vi "MGCC_FntStaMach_Visitualization_OpalRT_demo.vi"() -> ()   [LabVIEW 2016]
panel:
  out "3":cluster{dbl[], dbl[]}(graph)
  in  "S1011-STATUS-CTRL":dbl
  in  "S0910-STATUS-CTRL":dbl
  in  "S0709-STATUS-CTRL":dbl
  in  "S0708-STATUS-CTRL":dbl
  in  "S0405-STATUS-CTRL":dbl
  in  "S0307-STATUS-CTRL":dbl
  in  "S0304-STATUS-CTRL":dbl
  in  "S0203-STATUS-CTRL":dbl
  out "7":cluster{dbl[], dbl[]}(graph)
  out "10":cluster{dbl[], dbl[]}(graph)
  out "13":cluster{dbl[], dbl[]}(graph)
  out "14":cluster{dbl[], dbl[]}(graph)
  out "6":cluster{dbl[], dbl[]}(graph)
  out "1":cluster{dbl[], dbl[]}(graph)
  in  "Tab Control 2":T1(tab)
  out "Loads Power":dbl(graph)
  out "Loads Power":dbl(graph)
  out "Loads Power":dbl(graph)
  out "Loads Power":dbl(graph)
  out "Loads Power":dbl(graph)
  out "Loads Power":dbl(graph)
  out "Loads Power":dbl(graph)
  out "Loads Power":dbl(graph)
  out "Loads Power":dbl(graph)
  in  "Tab Control":T1(tab)
  out "Voltage":dbl(graph)
  out "Voltage":dbl(graph)
  out "Voltage":dbl(graph)
  out "Voltage":dbl(graph)
  out "Voltage":dbl(graph)
  out "Voltage":dbl(graph)
  out "Voltage":dbl(graph)
  out "Voltage":dbl(graph)
  out "Voltage":dbl(graph)
  out "Data Acquisition":bool
  out "Reactive power control":bool
  out "Active power control":bool
  out "Resynchronization":bool
  out "Communication":bool
  out "Data Acquisition":bool
  out "Reactive power control":bool
  out "Active power control":bool
  out "Resynchronization":bool
  out "Communication":bool
  in  "Island 3":bool
  in  "Island 2":bool
  in  "Island":bool
  in  "Ready for STD":bool
  in  "Recon cmd":bool
  in  "BKS cmd":bool
  in  "island cmd":bool
  out "Angle Difference 4":dbl
  out "Angle Difference 3":dbl
  out "Angle Difference 2":dbl
  out "Angle Difference 1":dbl
  out "BESS LC":bool
  out "PV LC":bool
  out "Model Mgmt.":bool
  out "PV Forecasting":bool
  out "Load Forecasting":bool
  out "PQ Balance":bool
  out "Black Start":bool
  out "Data Logging":bool
  out "Communication":bool
  out "State Estimation":bool
  out "Energy Mgmt.":bool
  out "SOC Tank":dbl(slide) scale=0.0..1.0
  out "S1114":bool
  out "S1011":bool
  out "S1012":bool
  out "S1013":bool
  out "S0910":bool
  out "S0708":bool
  out "S0709":bool
  out "S0307":bool
  out "S0304":bool
  out "S0406":bool
  out "S0405":bool
  out "S0203":bool
  out "S0102":bool
  out "W11":bool
  out "W13":bool
  out "W5":bool
  out "W8":bool
  out "L11":bool
  out "W12":bool
  out "L10":bool
  out "L7":bool
  out "L9":bool
  out "W7":bool
  out "W14":bool
  out "L8":bool
  out "L4":bool
  out "L5":bool
  out "W6":bool
  out "W3":bool
  out "L3":bool
  out "W2":bool
  out "L2":bool
  out "W1":bool
  out "Battery Output":dbl format="%#_6f"
  out "Battery SOC":dbl format="%#_6f"
  in  "PV-12":dbl(slide) scale=0.0..2.0
  out "PV Power Output":dbl format="%#_6f"
  out "PV Forecast":dbl[](graph)
  out "W4":bool
  out "Current State":string
  out "Sources Power":T2(graph)
  out "Frequency":T3(graph)
  out "W9":bool
  # "Title"
  # "G-6"
  # "Microgrid Local\nController 1"
  # "G-14"
  # "Microgrid Local\nController 2"
  # "Microgrid Central\nController"
  # "G-1"
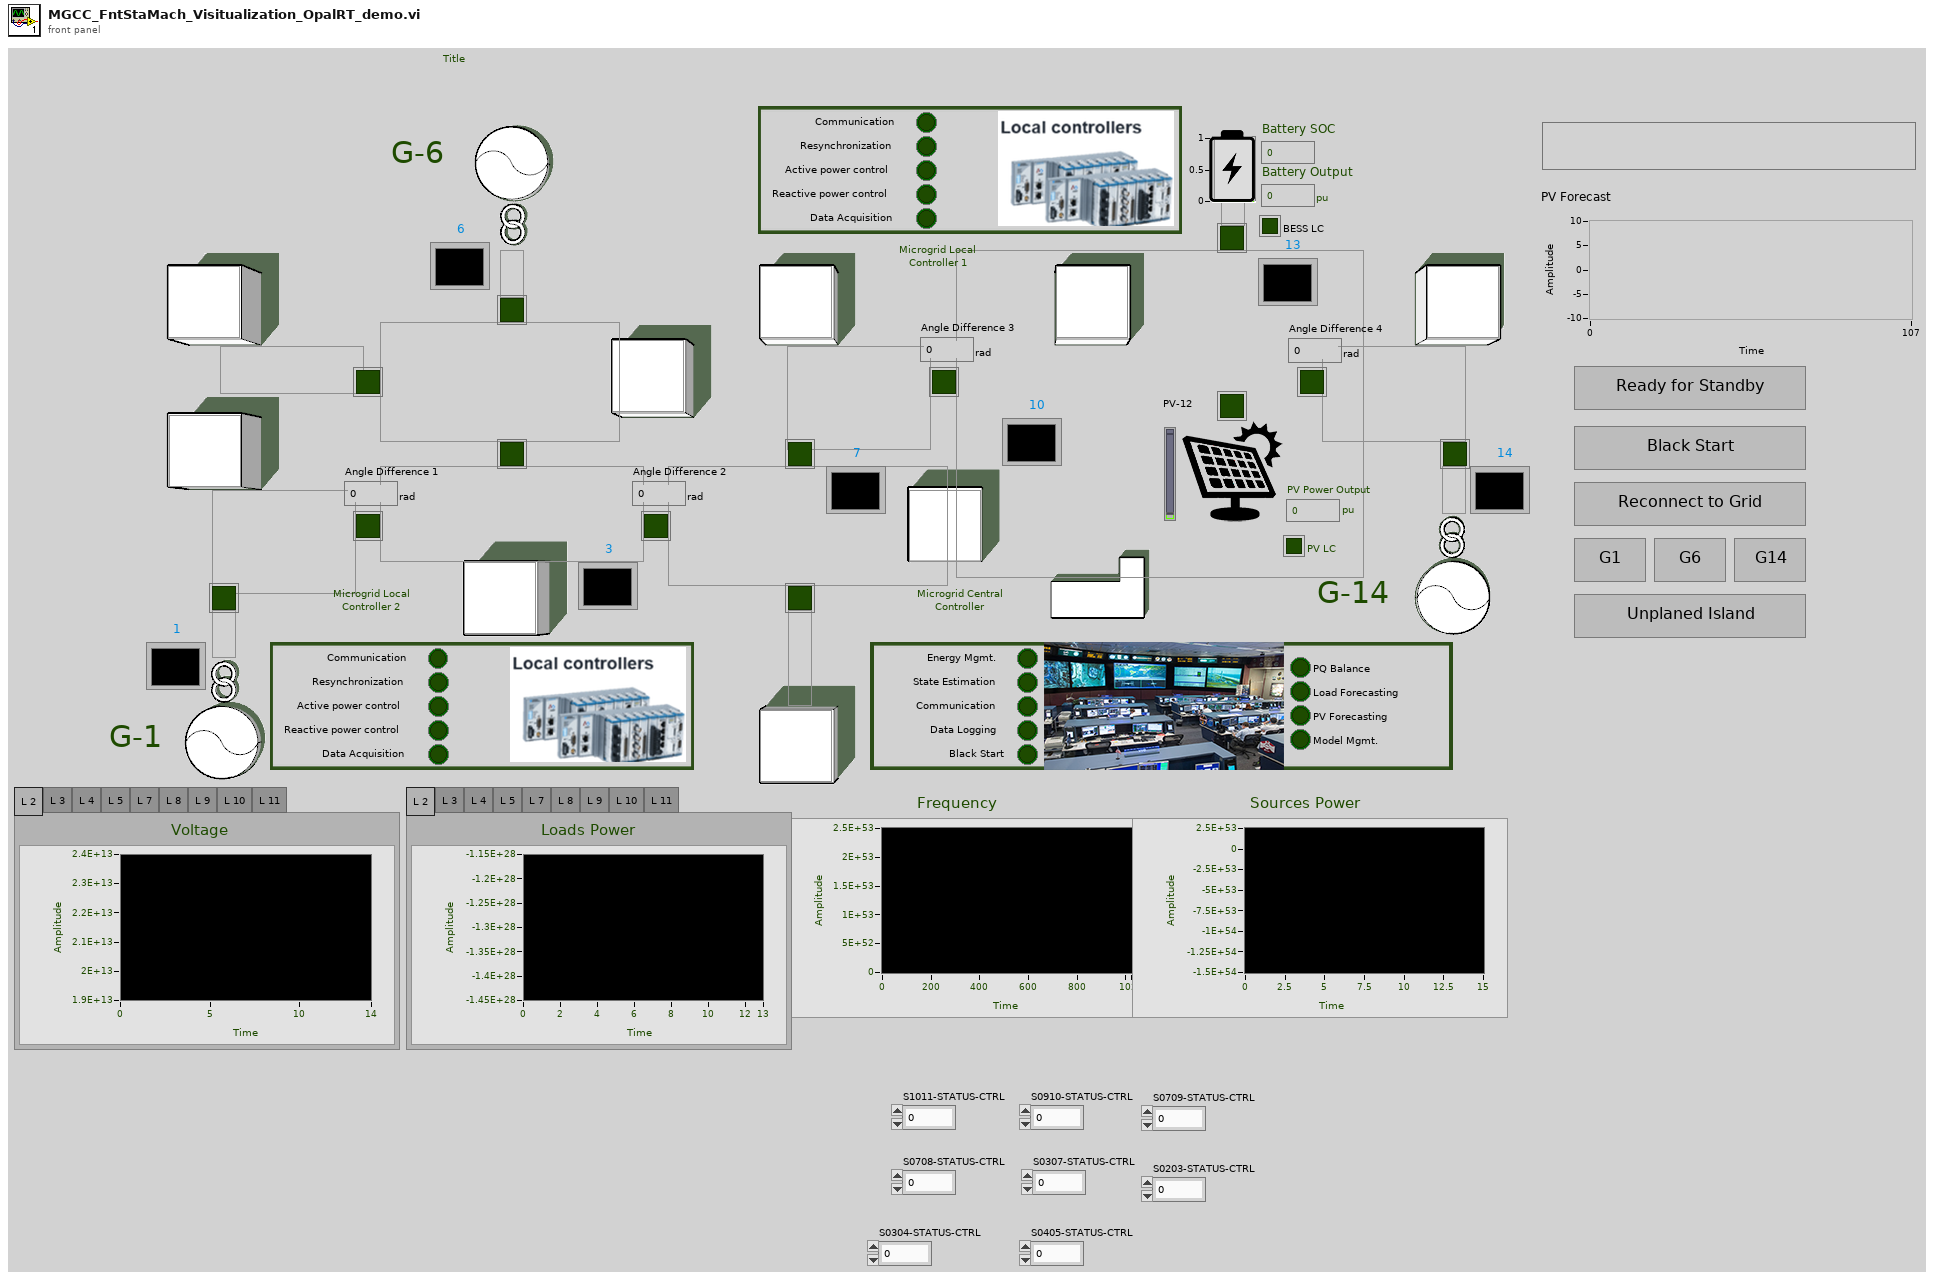
[diagram p1: front panel]
types:
  T1 = enum32{"L 2", "L 3", "L 4", "L 5", "L 7", "L 8", "L 9", "L 10", "L 11"}
  T2 = cluster{"Double":dbl, "Double":dbl, "Double":dbl, "Double":dbl, "Double":dbl}
  T3 = cluster{"Double":dbl, "Double":dbl, "Double":dbl, "Double":dbl}
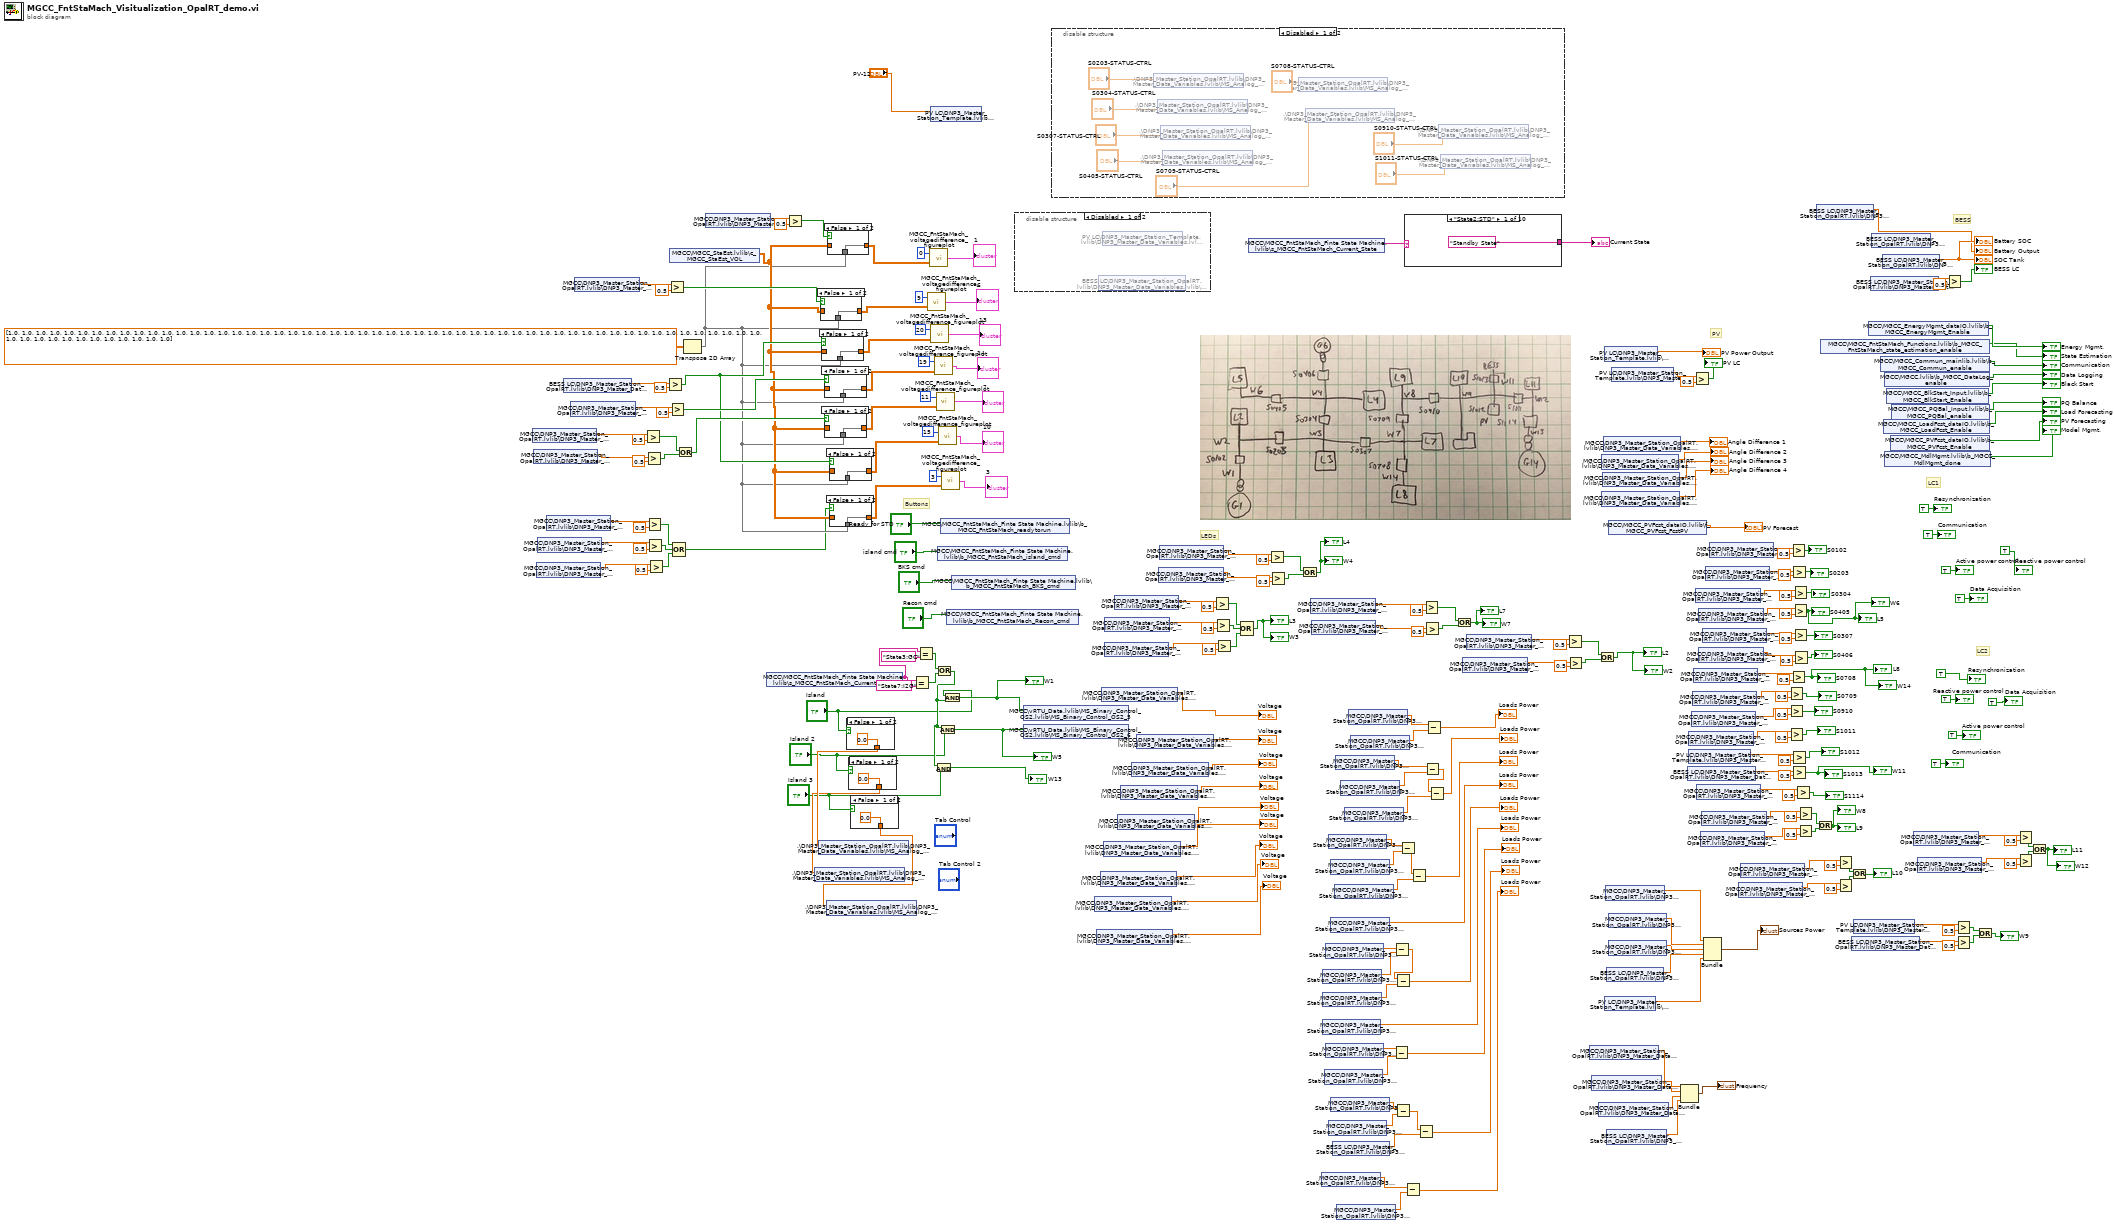
[diagram p0: block diagram]
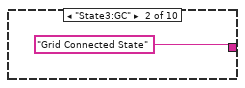
[diagram p2: hidden frame]
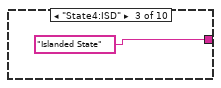
[diagram p3: hidden frame]
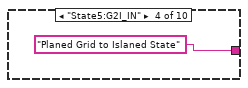
[diagram p4: hidden frame]
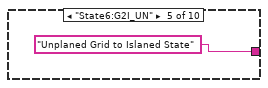
[diagram p5: hidden frame]
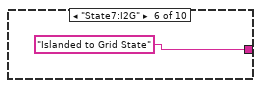
[diagram p6: hidden frame]
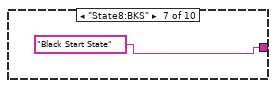
[diagram p7: hidden frame]
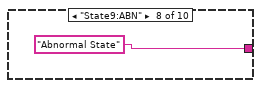
[diagram p8: hidden frame]
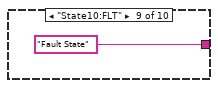
[diagram p9: hidden frame]
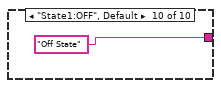
[diagram p10: hidden frame]
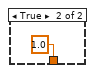
[diagram p12: hidden frame]
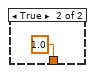
[diagram p13: hidden frame]
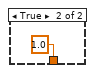
[diagram p14: hidden frame]
diagram:
  # "LC1"
  # "LC2"
  # "PV"
  # "BESS"
  # "Buttons"
  # "LEDs"
  n1 = shared-variable "MGCC\\DNP3_Master_Station_OpalRT.lvlib\\DNP3_Master_Data_Variables.lvlib\\MS_Analog_Status.lvlib\\S0307-status"() -> (w29:dbl)  [unwired: 1 in, 1 out]
  n2 = shared-variable "MGCC\\DNP3_Master_Station_OpalRT.lvlib\\DNP3_Master_Data_Variables.lvlib\\MS_Analog_Status.lvlib\\S0709-status"() -> (w28:dbl)  [unwired: 1 in, 1 out]
  n3 = shared-variable "MGCC\\DNP3_Master_Station_OpalRT.lvlib\\DNP3_Master_Data_Variables.lvlib\\MS_Analog_Status.lvlib\\S0307-status"() -> (w15:dbl)  [unwired: 1 in, 1 out]
  n4 = shared-variable "MGCC\\DNP3_Master_Station_OpalRT.lvlib\\DNP3_Master_Data_Variables.lvlib\\MS_Analog_Status.lvlib\\S0304-status"() -> (w16:dbl)  [unwired: 1 in, 1 out]
  n5 = shared-variable "MGCC\\DNP3_Master_Station_OpalRT.lvlib\\DNP3_Master_Data_Variables.lvlib\\MS_Analog_Status.lvlib\\S0203-status"() -> (w17:dbl)  [unwired: 1 in, 1 out]
  n6 = shared-variable "BESS LC\\DNP3_Master_Station_OpalRT.lvlib\\DNP3_Master_Data_Variables.lvlib\\MS_Analog_Status.lvlib\\BESS-STATUS"() -> (w41:dbl)  [unwired: 1 in, 1 out]
  n7 = shared-variable "MGCC\\DNP3_Master_Station_OpalRT.lvlib\\DNP3_Master_Data_Variables.lvlib\\MS_Analog_Status.lvlib\\S1114-status"() -> (w35:dbl)  [unwired: 1 in, 1 out]
  n8 = shared-variable "MGCC\\DNP3_Master_Station_OpalRT.lvlib\\DNP3_Master_Data_Variables.lvlib\\MS_Analog_Status.lvlib\\S0406-status"() -> (w44:dbl)  [unwired: 1 in, 1 out]
  n9 = Greater?(x=w29, y=0.5) -> (0:w31:bool)
  n10 = Greater?(x=w28, y=0.5) -> (0:w30:bool)
  n11 = Greater?(x=w17, y=0.5) -> (0:w14:bool)
  n12 = Greater?(x=w16, y=0.5) -> (0:w13:bool)
  n13 = Greater?(x=w15, y=0.5) -> (0:w12:bool)
  n14 = Greater?(x=w41, y=0.5) -> (0:w26:bool)
  n15 = Greater?(x=w44, y=0.5) -> (0:w43:bool)
  n16 = Greater?(x=w35, y=0.5) -> (0:w34:bool)
  n17 = shared-variable "MGCC\\MGCC_StaEst.lvlib\\c_MGCC_StaEst_VOL"() -> (w22:cdb[][])  [unwired: 1 in, 1 out]
  n18 = Compound Arithmetic op=OR(w14, w13, w12) -> (w11:bool)
  n19 = Or(x=w31, y=w30) -> (x .or. y?=w27:bool)
  n20 = Transpose 2D Array(2D array=dbl[][] [[1.0, 1.0, 1.0, 1.0, 1.0, 1.0, 1.0, 1.0, 1.0, 1.0, 1.0, 1.0, 1.0, 1.0, 1.0, 1.0, 1.0, 1.0, 1.0, 1.0, 1.0, 1.0], [1.0, 1.0, 1.0, 1.0, 1.0, 1.0, 1.0, 1.0, 1.0, 1.0, 1.0, 1.0, 1.0, 1.0, 1.0, 1.0, 1.0, 1.0, 1.0, 1.0, 1.0, 1.0], [1.0, 1.0, 1.0, 1.0, 1.0, 1.0, 1.0, 1.0, 1.0, 1.0, 1.0, 1.0, 1.0, 1.0, 1.0, 1.0, 1.0, 1.0, 1.0, 1.0, 1.0, 1.0]] ("lower limit")) -> (transposed array=w21:dbl[][])
  n21 = shared-variable "MGCC\\DNP3_Master_Station_OpalRT.lvlib\\DNP3_Master_Data_Variables.lvlib\\MS_Analog_Status.lvlib\\S0102-status"() -> (w48:dbl)  [unwired: 1 in, 1 out]
  n22 = shared-variable "MGCC\\MGCC_FntStaMach_Finte State Machine.lvlib\\s_MGCC_FntStaMach_Current_State"() -> (w64:string)  [unwired: 1 in, 1 out]
  n23 = Greater?(x=w48, y=0.5) -> (0:w47:bool)
  n24 = case shown="False" w43 {
    tunnel: w22 -> [_ w259]
    tunnel: [w258 w259] -> w46
    tunnel: w21 -> [w258 _]
    frame False {
    }
    frame True {
    }
  }
  n25 = case shown="False" w26 {
    tunnel: w22 -> [_ w261]
    tunnel: [w260 w261] -> w40
    tunnel: w21 -> [w260 _]
    frame False {
    }
    frame True {
    }
  }
  n26 = case shown="False" w34 {
    tunnel: w22 -> [_ w263]
    tunnel: [w262 w263] -> w39
    tunnel: w21 -> [w262 _]
    frame False {
    }
    frame True {
    }
  }
  n27 = case shown="False" w27 {
    tunnel: w22 -> [_ w265]
    tunnel: [w264 w265] -> w38
    tunnel: w21 -> [w264 _]
    frame False {
    }
    frame True {
    }
  }
  n28 = case shown="False" w47 {
    tunnel: w22 -> [_ w267]
    tunnel: [w266 w267] -> w50
    tunnel: w21 -> [w266 _]
    frame False {
    }
    frame True {
    }
  }
  n29 = case shown="False" w26 {
    tunnel: w22 -> [_ w269]
    tunnel: [w268 w269] -> w37
    tunnel: w21 -> [w268 _]
    frame False {
    }
    frame True {
    }
  }
  n30 = case shown="False" w11 {
    tunnel: w22 -> [_ w271]
    tunnel: [w270 w271] -> w23
    tunnel: w21 -> [w270 _]
    frame False {
    }
    frame True {
    }
  }
  n31 = case shown="False" "Island" {
    tunnel: [0.0 1.0] -> w8
    frame False {
    }
    frame True {
    }
  }
  n32 = shared-variable ".\\DNP3_Master_Station_OpalRT.lvlib\\DNP3_Master_Data_Variables.lvlib\\MS_Analog_Control.lvlib\\S0102-STATUS-CTRL"(w8) -> ()  [unwired: 1 in, 1 out]
  n33 = case shown="False" "Island 2" {
    tunnel: [0.0 1.0] -> w6
    frame False {
    }
    frame True {
    }
  }
  n34 = shared-variable ".\\DNP3_Master_Station_OpalRT.lvlib\\DNP3_Master_Data_Variables.lvlib\\MS_Analog_Control.lvlib\\S0406-STATUS-CTRL"(w6) -> ()  [unwired: 1 in, 1 out]
  n35 = case shown="False" "Island 3" {
    tunnel: [0.0 1.0] -> w4
    frame False {
    }
    frame True {
    }
  }
  n36 = shared-variable ".\\DNP3_Master_Station_OpalRT.lvlib\\DNP3_Master_Data_Variables.lvlib\\MS_Analog_Control.lvlib\\S1114-STATUS-CTRL"(w4) -> ()  [unwired: 1 in, 1 out]
  n37 = Equal?(x=w64, y="State7:I2G") -> (x = y?=w229:bool)
  n38 = Equal?(x=w64, y="State3:GC") -> (x = y?=w228:bool)
  n39 = call "MGCC_FntStaMach_voltagedifference_figureplot.vi"("array"=w46, "index (row)"=9) -> ("output cluster"=→"6":cluster{dbl[], dbl[]})
  n40 = call "MGCC_FntStaMach_voltagedifference_figureplot.vi"("array"=w50, "index (row)"=0) -> ("output cluster"=→"1":cluster{dbl[], dbl[]})
  n41 = shared-variable "PV LC\\DNP3_Master_Station_Template.lvlib\\DNP3_Master_Data_Variables.lvlib\\MS_Analog_Control.lvlib\\PV-APC"("PV-12") -> ()  [unwired: 1 in, 1 out]
  n42 = call "MGCC_FntStaMach_voltagedifference_figureplot.vi"("array"=w40, "index (row)"=20) -> ("output cluster"=→"13":cluster{dbl[], dbl[]})
  n43 = call "MGCC_FntStaMach_voltagedifference_figureplot.vi"("array"=w39, "index (row)"=19) -> ("output cluster"=→"14":cluster{dbl[], dbl[]})
  n44 = Or(x=w228, y=w229) -> (x .or. y?=w227:bool)
  n45 = And(x=w227, y="Island 3") -> (x .and. y?=→"W13":bool)
  n46 = call "MGCC_FntStaMach_voltagedifference_figureplot.vi"("array"=w38, "index (row)"=11) -> ("output cluster"=→"7":cluster{dbl[], dbl[]})
  n47 = shared-variable "MGCC\\MGCC_FntStaMach_Finte State Machine.lvlib\\b_MGCC_FntStaMach_island_cmd"("island cmd") -> ()  [unwired: 1 in, 1 out]
  n48 = call "MGCC_FntStaMach_voltagedifference_figureplot.vi"("array"=w37, "index (row)"=15) -> ("output cluster"=→"10":cluster{dbl[], dbl[]})
  n49 = And(x=w227, y="Island 2") -> (x .and. y?=w225:bool)
  "W5" <- w225
  n50 = shared-variable "MGCC\\MGCC_FntStaMach_Finte State Machine.lvlib\\b_MGCC_FntStaMach_readytorun"("Ready for STD") -> ()  [unwired: 1 in, 1 out]
  n51 = call "MGCC_FntStaMach_voltagedifference_figureplot.vi"("array"=w23, "index (row)"=3) -> ("output cluster"=→"3":cluster{dbl[], dbl[]})
  n52 = And(x="Island", y=w227) -> (x .and. y?=w226:bool)
  "W1" <- w226
  n53 = shared-variable "MGCC\\MGCC_FntStaMach_Finte State Machine.lvlib\\b_MGCC_FntStaMach_Recon_cmd"("Recon cmd") -> ()  [unwired: 1 in, 1 out]
  n54 = shared-variable "MGCC\\MGCC_FntStaMach_Finte State Machine.lvlib\\b_MGCC_FntStaMach_BKS_cmd"("BKS cmd") -> ()  [unwired: 1 in, 1 out]
  n55 = disable-structure shown="Disabled" {
    frame Disabled {
      n56 = shared-variable "BESS LC\\DNP3_Master_Station_OpalRT.lvlib\\DNP3_Master_Data_Variables.lvlib\\MS_Analog_Control.lvlib\\BESS-STATUS-CTRL"() -> (w279:dbl)  [unwired: 1 in, 1 out]
      n57 = shared-variable "PV LC\\DNP3_Master_Station_Template.lvlib\\DNP3_Master_Data_Variables.lvlib\\MS_Analog_Control.lvlib\\PV-STATUS-CTRL"() -> (w278:dbl)  [unwired: 1 in, 1 out]
    }
    frame Enabled {
    }
  }
  n58 = shared-variable "MGCC\\vRTU_Data.lvlib\\MS_Binary_Control_OS2.lvlib\\MS_Binary_Control_OS2_5"(w226) -> ()  [unwired: 1 in, 1 out]
  n59 = shared-variable "MGCC\\vRTU_Data.lvlib\\MS_Binary_Control_OS2.lvlib\\MS_Binary_Control_OS2_6"(w225) -> ()  [unwired: 1 in, 1 out]
  n60 = disable-structure shown="Disabled" {
    frame Disabled {
      n61 = shared-variable ".\\DNP3_Master_Station_OpalRT.lvlib\\DNP3_Master_Data_Variables.lvlib\\MS_Analog_Control.lvlib\\S0203-STATUS-CTRL"("S0203-STATUS-CTRL") -> ()  [unwired: 1 in, 1 out]
      n62 = shared-variable ".\\DNP3_Master_Station_OpalRT.lvlib\\DNP3_Master_Data_Variables.lvlib\\MS_Analog_Control.lvlib\\S0304-STATUS-CTRL"("S0304-STATUS-CTRL") -> ()  [unwired: 1 in, 1 out]
      n63 = shared-variable ".\\DNP3_Master_Station_OpalRT.lvlib\\DNP3_Master_Data_Variables.lvlib\\MS_Analog_Control.lvlib\\S0307-STATUS-CTRL"("S0307-STATUS-CTRL") -> ()  [unwired: 1 in, 1 out]
      n64 = shared-variable ".\\DNP3_Master_Station_OpalRT.lvlib\\DNP3_Master_Data_Variables.lvlib\\MS_Analog_Control.lvlib\\S0405-STATUS-CTRL"("S0405-STATUS-CTRL") -> ()  [unwired: 1 in, 1 out]
      n65 = shared-variable ".\\DNP3_Master_Station_OpalRT.lvlib\\DNP3_Master_Data_Variables.lvlib\\MS_Analog_Control.lvlib\\S0708-STATUS-CTRL"("S0708-STATUS-CTRL") -> ()  [unwired: 1 in, 1 out]
      n66 = shared-variable ".\\DNP3_Master_Station_OpalRT.lvlib\\DNP3_Master_Data_Variables.lvlib\\MS_Analog_Control.lvlib\\S0709-STATUS-CTRL"("S0709-STATUS-CTRL") -> ()  [unwired: 1 in, 1 out]
      n67 = shared-variable ".\\DNP3_Master_Station_OpalRT.lvlib\\DNP3_Master_Data_Variables.lvlib\\MS_Analog_Control.lvlib\\S0910-STATUS-CTRL"("S0910-STATUS-CTRL") -> ()  [unwired: 1 in, 1 out]
      n68 = shared-variable ".\\DNP3_Master_Station_OpalRT.lvlib\\DNP3_Master_Data_Variables.lvlib\\MS_Analog_Control.lvlib\\S1011-STATUS-CTRL"("S1011-STATUS-CTRL") -> ()  [unwired: 1 in, 1 out]
    }
    frame Enabled {
    }
  }
  n69 = shared-variable "MGCC\\DNP3_Master_Station_OpalRT.lvlib\\DNP3_Master_Data_Variables.lvlib\\MS_Analog_Status.lvlib\\S0910-MAG-A-R"() -> (→"Voltage":dbl)  [unwired: 1 in, 1 out]
  n70 = shared-variable "MGCC\\DNP3_Master_Station_OpalRT.lvlib\\DNP3_Master_Data_Variables.lvlib\\MS_Analog_Status.lvlib\\S1011-MAG-A-R"() -> (→"Voltage":dbl)  [unwired: 1 in, 1 out]
  n71 = shared-variable "MGCC\\DNP3_Master_Station_OpalRT.lvlib\\DNP3_Master_Data_Variables.lvlib\\MS_Analog_Status.lvlib\\S0709-MAG-A-R"() -> (→"Voltage":dbl)  [unwired: 1 in, 1 out]
  n72 = shared-variable "MGCC\\DNP3_Master_Station_OpalRT.lvlib\\DNP3_Master_Data_Variables.lvlib\\MS_Analog_Status.lvlib\\S0102-MAG-A-R"() -> (→"Voltage":dbl)  [unwired: 1 in, 1 out]
  n73 = shared-variable "MGCC\\DNP3_Master_Station_OpalRT.lvlib\\DNP3_Master_Data_Variables.lvlib\\MS_Analog_Status.lvlib\\S0708-MAG-A-R"() -> (→"Voltage":dbl)  [unwired: 1 in, 1 out]
  n74 = shared-variable "MGCC\\DNP3_Master_Station_OpalRT.lvlib\\DNP3_Master_Data_Variables.lvlib\\MS_Analog_Status.lvlib\\S0307-status"() -> (w114:dbl)  [unwired: 1 in, 1 out]
  n75 = shared-variable "MGCC\\DNP3_Master_Station_OpalRT.lvlib\\DNP3_Master_Data_Variables.lvlib\\MS_Analog_Status.lvlib\\S0304-status"() -> (w115:dbl)  [unwired: 1 in, 1 out]
  n76 = shared-variable "MGCC\\DNP3_Master_Station_OpalRT.lvlib\\DNP3_Master_Data_Variables.lvlib\\MS_Analog_Status.lvlib\\S0203-status"() -> (w116:dbl)  [unwired: 1 in, 1 out]
  n77 = shared-variable "MGCC\\DNP3_Master_Station_OpalRT.lvlib\\DNP3_Master_Data_Variables.lvlib\\MS_Analog_Status.lvlib\\S0307-MAG-A-R"() -> (→"Voltage":dbl)  [unwired: 1 in, 1 out]
  n78 = shared-variable "MGCC\\DNP3_Master_Station_OpalRT.lvlib\\DNP3_Master_Data_Variables.lvlib\\MS_Analog_Status.lvlib\\S0405-MAG-A-R"() -> (→"Voltage":dbl)  [unwired: 1 in, 1 out]
  n79 = shared-variable "MGCC\\DNP3_Master_Station_OpalRT.lvlib\\DNP3_Master_Data_Variables.lvlib\\MS_Analog_Status.lvlib\\S0304-MAG-A-R"() -> (→"Voltage":dbl)  [unwired: 1 in, 1 out]
  n80 = shared-variable "MGCC\\DNP3_Master_Station_OpalRT.lvlib\\DNP3_Master_Data_Variables.lvlib\\MS_Analog_Status.lvlib\\S0203-MAG-A-R"() -> (→"Voltage":dbl)  [unwired: 1 in, 1 out]
  n81 = shared-variable "MGCC\\DNP3_Master_Station_OpalRT.lvlib\\DNP3_Master_Data_Variables.lvlib\\MS_Analog_Status.lvlib\\S0406-status"() -> (w104:dbl)  [unwired: 1 in, 1 out]
  n82 = shared-variable "MGCC\\DNP3_Master_Station_OpalRT.lvlib\\DNP3_Master_Data_Variables.lvlib\\MS_Analog_Status.lvlib\\S0304-status"() -> (w105:dbl)  [unwired: 1 in, 1 out]
  n83 = Greater?(x=w116, y=0.5) -> (0:w113:bool)
  n84 = Greater?(x=w115, y=0.5) -> (0:w112:bool)
  n85 = Greater?(x=w114, y=0.5) -> (0:w111:bool)
  n86 = Compound Arithmetic op=OR(w113, w112, w111) -> (→"L3" →"W3":bool)
  n87 = shared-variable "MGCC\\MGCC_FntStaMach_Finte State Machine.lvlib\\s_MGCC_FntStaMach_Current_State"() -> (w2:string)  [unwired: 1 in, 1 out]
  n88 = Greater?(x=w105, y=0.5) -> (0:w107:bool)
  n89 = Greater?(x=w104, y=0.5) -> (0:w106:bool)
  n90 = Or(x=w107, y=w106) -> (x .or. y?=→"W4" →"L4":bool)
  n91 = shared-variable "MGCC\\DNP3_Master_Station_OpalRT.lvlib\\DNP3_Master_Data_Variables.lvlib\\MS_Analog_Status.lvlib\\S0307-status"() -> (w98:dbl)  [unwired: 1 in, 1 out]
  n92 = shared-variable "MGCC\\DNP3_Master_Station_OpalRT.lvlib\\DNP3_Master_Data_Variables.lvlib\\MS_Analog_Status.lvlib\\S0709-status"() -> (w97:dbl)  [unwired: 1 in, 1 out]
  n93 = shared-variable "MGCC\\DNP3_Master_Station_OpalRT.lvlib\\DNP3_Master_Data_Variables.lvlib\\MS_Analog_Status.lvlib\\S1011-APF"() -> (w186:dbl)  [unwired: 1 in, 1 out]
  n94 = shared-variable "MGCC\\DNP3_Master_Station_OpalRT.lvlib\\DNP3_Master_Data_Variables.lvlib\\MS_Analog_Status.lvlib\\S0708-APF"() -> (→"Loads Power":dbl)  [unwired: 1 in, 1 out]
  n95 = shared-variable "MGCC\\DNP3_Master_Station_OpalRT.lvlib\\DNP3_Master_Data_Variables.lvlib\\MS_Analog_Status.lvlib\\S0708-APF"() -> (w199:dbl)  [unwired: 1 in, 1 out]
  n96 = shared-variable "MGCC\\DNP3_Master_Station_OpalRT.lvlib\\DNP3_Master_Data_Variables.lvlib\\MS_Analog_Status.lvlib\\S0709-APF"() -> (w197:dbl)  [unwired: 1 in, 1 out]
  n97 = shared-variable "MGCC\\DNP3_Master_Station_OpalRT.lvlib\\DNP3_Master_Data_Variables.lvlib\\MS_Analog_Status.lvlib\\S0910-APF"() -> (w193:dbl)  [unwired: 1 in, 1 out]
  n98 = shared-variable "MGCC\\DNP3_Master_Station_OpalRT.lvlib\\DNP3_Master_Data_Variables.lvlib\\MS_Analog_Status.lvlib\\S0307-APF"() -> (w200:dbl)  [unwired: 1 in, 1 out]
  n99 = shared-variable "MGCC\\DNP3_Master_Station_OpalRT.lvlib\\DNP3_Master_Data_Variables.lvlib\\MS_Analog_Status.lvlib\\S0709-APF"() -> (w194:dbl)  [unwired: 1 in, 1 out]
  n100 = shared-variable "MGCC\\DNP3_Master_Station_OpalRT.lvlib\\DNP3_Master_Data_Variables.lvlib\\MS_Analog_Status.lvlib\\S0304-APF"() -> (w206:dbl)  [unwired: 1 in, 1 out]
  n101 = shared-variable "MGCC\\DNP3_Master_Station_OpalRT.lvlib\\DNP3_Master_Data_Variables.lvlib\\MS_Analog_Status.lvlib\\S1011-APF"() -> (w190:dbl)  [unwired: 1 in, 1 out]
  n102 = shared-variable "MGCC\\DNP3_Master_Station_OpalRT.lvlib\\DNP3_Master_Data_Variables.lvlib\\MS_Analog_Status.lvlib\\S0405-APF"() -> (w205:dbl)  [unwired: 1 in, 1 out]
  n103 = shared-variable "MGCC\\DNP3_Master_Station_OpalRT.lvlib\\DNP3_Master_Data_Variables.lvlib\\MS_Analog_Status.lvlib\\S0405-APF"() -> (→"Loads Power":dbl)  [unwired: 1 in, 1 out]
  n104 = shared-variable "MGCC\\DNP3_Master_Station_OpalRT.lvlib\\DNP3_Master_Data_Variables.lvlib\\MS_Analog_Status.lvlib\\S0910-APF"() -> (w191:dbl)  [unwired: 1 in, 1 out]
  n105 = shared-variable "BESS LC\\DNP3_Master_Station_OpalRT.lvlib\\DNP3_Master_Data_Variables.lvlib\\MS_Analog_Status.lvlib\\BESS-APO"() -> (w188:dbl)  [unwired: 1 in, 1 out]
  n106 = shared-variable "MGCC\\DNP3_Master_Station_OpalRT.lvlib\\DNP3_Master_Data_Variables.lvlib\\MS_Analog_Status.lvlib\\S0406-APF"() -> (w203:dbl)  [unwired: 1 in, 1 out]
  n107 = shared-variable "MGCC\\DNP3_Master_Station_OpalRT.lvlib\\DNP3_Master_Data_Variables.lvlib\\MS_Analog_Status.lvlib\\S0203-APF"() -> (w211:dbl)  [unwired: 1 in, 1 out]
  n108 = shared-variable "MGCC\\DNP3_Master_Station_OpalRT.lvlib\\DNP3_Master_Data_Variables.lvlib\\MS_Analog_Status.lvlib\\S1114-APF"() -> (w185:dbl)  [unwired: 1 in, 1 out]
  n109 = shared-variable "MGCC\\DNP3_Master_Station_OpalRT.lvlib\\DNP3_Master_Data_Variables.lvlib\\MS_Analog_Status.lvlib\\S0304-APF"() -> (w210:dbl)  [unwired: 1 in, 1 out]
  n110 = shared-variable "MGCC\\DNP3_Master_Station_OpalRT.lvlib\\DNP3_Master_Data_Variables.lvlib\\MS_Analog_Status.lvlib\\S0307-APF"() -> (w208:dbl)  [unwired: 1 in, 1 out]
  n111 = shared-variable "MGCC\\DNP3_Master_Station_OpalRT.lvlib\\DNP3_Master_Data_Variables.lvlib\\MS_Analog_Status.lvlib\\S0102-APF"() -> (w214:dbl)  [unwired: 1 in, 1 out]
  n112 = shared-variable "MGCC\\DNP3_Master_Station_OpalRT.lvlib\\DNP3_Master_Data_Variables.lvlib\\MS_Analog_Status.lvlib\\S0203-APF"() -> (w213:dbl)  [unwired: 1 in, 1 out]
  n113 = Subtract(x=w194, y=w193) -> (x-y=→"Loads Power":dbl)
  n114 = Subtract(x=w200, y=w199) -> (x-y=w198:dbl)
  n115 = Subtract(x=w198, y=w197) -> (x-y=→"Loads Power":dbl)
  n116 = Subtract(x=w191, y=w190) -> (x-y=w189:dbl)
  n117 = Subtract(x=w206, y=w205) -> (x-y=w204:dbl)
  n118 = case shown="\"State2:STD\"" w2 {
    tunnel: ["Standby State" "Grid Connected State" "Islanded State" "Planed Grid to Islaned State" "Unplaned Grid to Islaned State" "Islanded to Grid State" "Black Start State" "Abnormal State" "Fault State" "Off State"] -> w1
    frame "State2:STD" {
    }
    frame "State3:GC" {
    }
    frame "State4:ISD" {
    }
    frame "State5:G2I_IN" {
    }
    frame "State6:G2I_UN" {
    }
    frame "State7:I2G" {
    }
    frame "State8:BKS" {
    }
    frame "State9:ABN" {
    }
    frame "State10:FLT" {
    }
    frame "State1:OFF", Default {
    }
  }
  "Current State" <- w1
  n119 = Subtract(x=w186, y=w185) -> (x-y=→"Loads Power":dbl)
  n120 = Subtract(x=w204, y=w203) -> (x-y=→"Loads Power":dbl)
  n121 = Subtract(x=w189, y=w188) -> (x-y=→"Loads Power":dbl)
  n122 = Greater?(x=w98, y=0.5) -> (0:w100:bool)
  n123 = Greater?(x=w97, y=0.5) -> (0:w99:bool)
  n124 = Subtract(x=w211, y=w210) -> (x-y=w209:dbl)
  n125 = Subtract(x=w214, y=w213) -> (x-y=→"Loads Power":dbl)
  n126 = Subtract(x=w209, y=w208) -> (x-y=→"Loads Power":dbl)
  n127 = Or(x=w100, y=w99) -> (x .or. y?=→"W7" →"L7":bool)
  n128 = shared-variable "MGCC\\DNP3_Master_Station_OpalRT.lvlib\\DNP3_Master_Data_Variables.lvlib\\MS_Analog_Status.lvlib\\S0203-status"() -> (w123:dbl)  [unwired: 1 in, 1 out]
  n129 = shared-variable "MGCC\\DNP3_Master_Station_OpalRT.lvlib\\DNP3_Master_Data_Variables.lvlib\\MS_Analog_Status.lvlib\\S0102-status"() -> (w124:dbl)  [unwired: 1 in, 1 out]
  n130 = Greater?(x=w124, y=0.5) -> (0:w122:bool)
  n131 = Greater?(x=w123, y=0.5) -> (0:w121:bool)
  n132 = shared-variable "MGCC\\DNP3_Master_Station_OpalRT.lvlib\\DNP3_Master_Data_Variables.lvlib\\MS_Analog_Status.lvlib\\S0102-FREQ-L"() -> (w183:dbl)  [unwired: 1 in, 1 out]
  n133 = shared-variable "MGCC\\DNP3_Master_Station_OpalRT.lvlib\\DNP3_Master_Data_Variables.lvlib\\MS_Analog_Status.lvlib\\S0406-FREQ-R"() -> (w182:dbl)  [unwired: 1 in, 1 out]
  n134 = Or(x=w122, y=w121) -> (x .or. y?=→"L2" →"W2":bool)
  n135 = shared-variable "MGCC\\DNP3_Master_Station_OpalRT.lvlib\\DNP3_Master_Data_Variables.lvlib\\MS_Analog_Status.lvlib\\S1114-FREQ-R"() -> (w181:dbl)  [unwired: 1 in, 1 out]
  n136 = shared-variable "MGCC\\DNP3_Master_Station_OpalRT.lvlib\\DNP3_Master_Data_Variables.lvlib\\MS_Analog_Status.lvlib\\S0307-ANG-DIFF"() -> (→"Angle Difference 2":dbl)  [unwired: 1 in, 1 out]
  n137 = shared-variable "MGCC\\DNP3_Master_Station_OpalRT.lvlib\\DNP3_Master_Data_Variables.lvlib\\MS_Analog_Status.lvlib\\S1011-ANG-DIFF"() -> (→"Angle Difference 4":dbl)  [unwired: 1 in, 1 out]
  n138 = shared-variable "MGCC\\DNP3_Master_Station_OpalRT.lvlib\\DNP3_Master_Data_Variables.lvlib\\MS_Analog_Status.lvlib\\S0910-ANG-DIFF"() -> (→"Angle Difference 3":dbl)  [unwired: 1 in, 1 out]
  n139 = shared-variable "MGCC\\DNP3_Master_Station_OpalRT.lvlib\\DNP3_Master_Data_Variables.lvlib\\MS_Analog_Status.lvlib\\S0203-ANG-DIFF"() -> (→"Angle Difference 1":dbl)  [unwired: 1 in, 1 out]
  n140 = shared-variable "PV LC\\DNP3_Master_Station_Template.lvlib\\DNP3_Master_Data_Variables.lvlib\\MS_Analog_Status.lvlib\\PV-MAG"() -> (→"PV Power Output":dbl)  [unwired: 1 in, 1 out]
  n141 = shared-variable "PV LC\\DNP3_Master_Station_Template.lvlib\\DNP3_Master_Data_Variables.lvlib\\MS_Analog_Status.lvlib\\PV-APO"() -> (w174:dbl)  [unwired: 1 in, 1 out]
  n142 = shared-variable "MGCC\\DNP3_Master_Station_OpalRT.lvlib\\DNP3_Master_Data_Variables.lvlib\\MS_Analog_Status.lvlib\\S0102-APF"() -> (w178:dbl)  [unwired: 1 in, 1 out]
  n143 = shared-variable "BESS LC\\DNP3_Master_Station_OpalRT.lvlib\\DNP3_Master_Data_Variables.lvlib\\MS_Analog_Status.lvlib\\BESS-APO"() -> (w175:dbl)  [unwired: 1 in, 1 out]
  n144 = shared-variable "BESS LC\\DNP3_Master_Station_OpalRT.lvlib\\DNP3_Master_Data_Variables.lvlib\\MS_Analog_Status.lvlib\\BESS-FREQ"() -> (w180:dbl)  [unwired: 1 in, 1 out]
  n145 = shared-variable "MGCC\\MGCC_PVFcst_dataIO.lvlib\\f_MGCC_PVFcst_FcstPV"() -> (→"PV Forecast":dbl[])  [unwired: 1 in, 1 out]
  n146 = shared-variable "MGCC\\DNP3_Master_Station_OpalRT.lvlib\\DNP3_Master_Data_Variables.lvlib\\MS_Analog_Status.lvlib\\S0406-APF"() -> (w177:dbl)  [unwired: 1 in, 1 out]
  n147 = shared-variable "MGCC\\DNP3_Master_Station_OpalRT.lvlib\\DNP3_Master_Data_Variables.lvlib\\MS_Analog_Status.lvlib\\S1114-APF"() -> (w176:dbl)  [unwired: 1 in, 1 out]
  n148 = shared-variable "PV LC\\DNP3_Master_Station_Template.lvlib\\DNP3_Master_Data_Variables.lvlib\\MS_Analog_Status.lvlib\\PV-STATUS"() -> (w242:dbl)  [unwired: 1 in, 1 out]
  n149 = Bundle("Double"=w183, "Double"=w182, "Double"=w181, "Double"=w180) -> (→"Frequency":T3)  [unwired: 1 in]
  n150 = shared-variable "BESS LC\\DNP3_Master_Station_OpalRT.lvlib\\DNP3_Master_Data_Variables.lvlib\\MS_Analog_Status.lvlib\\BESS-STATUS"() -> (w127:dbl)  [unwired: 1 in, 1 out]
  n151 = shared-variable "MGCC\\DNP3_Master_Station_OpalRT.lvlib\\DNP3_Master_Data_Variables.lvlib\\MS_Analog_Status.lvlib\\S1011-status"() -> (w133:dbl)  [unwired: 1 in, 1 out]
  n152 = shared-variable "PV LC\\DNP3_Master_Station_Template.lvlib\\DNP3_Master_Data_Variables.lvlib\\MS_Analog_Status.lvlib\\PV-STATUS"() -> (w129:dbl)  [unwired: 1 in, 1 out]
  n153 = shared-variable "MGCC\\DNP3_Master_Station_OpalRT.lvlib\\DNP3_Master_Data_Variables.lvlib\\MS_Analog_Status.lvlib\\S0910-status"() -> (w135:dbl)  [unwired: 1 in, 1 out]
  n154 = shared-variable "MGCC\\DNP3_Master_Station_OpalRT.lvlib\\DNP3_Master_Data_Variables.lvlib\\MS_Analog_Status.lvlib\\S0709-status"() -> (w141:dbl)  [unwired: 1 in, 1 out]
  n155 = Greater?(x=w242, y=0.5) -> (0:→"PV LC":bool)
  n156 = shared-variable "MGCC\\DNP3_Master_Station_OpalRT.lvlib\\DNP3_Master_Data_Variables.lvlib\\MS_Analog_Status.lvlib\\S0708-status"() -> (w142:dbl)  [unwired: 1 in, 1 out]
  n157 = shared-variable "MGCC\\DNP3_Master_Station_OpalRT.lvlib\\DNP3_Master_Data_Variables.lvlib\\MS_Analog_Status.lvlib\\S0304-status"() -> (w154:dbl)  [unwired: 1 in, 1 out]
  n158 = shared-variable "MGCC\\DNP3_Master_Station_OpalRT.lvlib\\DNP3_Master_Data_Variables.lvlib\\MS_Analog_Status.lvlib\\S1114-status"() -> (w131:dbl)  [unwired: 1 in, 1 out]
  n159 = shared-variable "MGCC\\DNP3_Master_Station_OpalRT.lvlib\\DNP3_Master_Data_Variables.lvlib\\MS_Analog_Status.lvlib\\S0405-status"() -> (w147:dbl)  [unwired: 1 in, 1 out]
  n160 = shared-variable "MGCC\\DNP3_Master_Station_OpalRT.lvlib\\DNP3_Master_Data_Variables.lvlib\\MS_Analog_Status.lvlib\\S0406-status"() -> (w144:dbl)  [unwired: 1 in, 1 out]
  n161 = shared-variable "MGCC\\DNP3_Master_Station_OpalRT.lvlib\\DNP3_Master_Data_Variables.lvlib\\MS_Analog_Status.lvlib\\S0910-status"() -> (w91:dbl)  [unwired: 1 in, 1 out]
  n162 = shared-variable "MGCC\\DNP3_Master_Station_OpalRT.lvlib\\DNP3_Master_Data_Variables.lvlib\\MS_Analog_Status.lvlib\\S0709-status"() -> (w92:dbl)  [unwired: 1 in, 1 out]
  n163 = shared-variable "MGCC\\DNP3_Master_Station_OpalRT.lvlib\\DNP3_Master_Data_Variables.lvlib\\MS_Analog_Status.lvlib\\S0307-status"() -> (w146:dbl)  [unwired: 1 in, 1 out]
  n164 = Bundle("Double"=w178, "Double"=w177, "Double"=w176, "Double"=w175, "Double"=w174) -> (→"Sources Power":T2)  [unwired: 1 in]
  n165 = shared-variable "MGCC\\DNP3_Master_Station_OpalRT.lvlib\\DNP3_Master_Data_Variables.lvlib\\MS_Analog_Status.lvlib\\S0203-status"() -> (w156:dbl)  [unwired: 1 in, 1 out]
  n166 = shared-variable "MGCC\\DNP3_Master_Station_OpalRT.lvlib\\DNP3_Master_Data_Variables.lvlib\\MS_Analog_Status.lvlib\\S0102-status"() -> (w161:dbl)  [unwired: 1 in, 1 out]
  n167 = shared-variable "MGCC\\DNP3_Master_Station_OpalRT.lvlib\\DNP3_Master_Data_Variables.lvlib\\MS_Analog_Status.lvlib\\S1011-status"() -> (w88:dbl)  [unwired: 1 in, 1 out]
  n168 = shared-variable "MGCC\\DNP3_Master_Station_OpalRT.lvlib\\DNP3_Master_Data_Variables.lvlib\\MS_Analog_Status.lvlib\\S0910-status"() -> (w87:dbl)  [unwired: 1 in, 1 out]
  n169 = Greater?(x=w141, y=0.5) -> (0:→"S0709":bool)
  n170 = Greater?(x=w135, y=0.5) -> (0:→"S0910":bool)
  n171 = Greater?(x=w133, y=0.5) -> (0:→"S1011":bool)
  n172 = Greater?(x=w161, y=0.5) -> (0:→"S0102":bool)
  n173 = Greater?(x=w142, y=0.5) -> (0:→"L8" →"W14" →"S0708":bool)
  n174 = Greater?(x=w156, y=0.5) -> (0:→"S0203":bool)
  n175 = Greater?(x=w129, y=0.5) -> (0:→"S1012":bool)
  n176 = Greater?(x=w127, y=0.5) -> (0:→"W11" →"S1013":bool)
  n177 = Greater?(x=w154, y=0.5) -> (0:→"S0304":bool)
  n178 = Greater?(x=w147, y=0.5) -> (0:→"W6" →"L5" →"S0405":bool)
  n179 = Greater?(x=w146, y=0.5) -> (0:→"S0307":bool)
  n180 = Greater?(x=w144, y=0.5) -> (0:→"S0406":bool)
  n181 = Greater?(x=w131, y=0.5) -> (0:→"S1114":bool)
  n182 = Greater?(x=w92, y=0.5) -> (0:w90:bool)
  n183 = Greater?(x=w91, y=0.5) -> (0:w89:bool)
  n184 = shared-variable "BESS LC\\DNP3_Master_Station_OpalRT.lvlib\\DNP3_Master_Data_Variables.lvlib\\MS_Analog_Status.lvlib\\BESS-APO"() -> (→"Battery Output":dbl)  [unwired: 1 in, 1 out]
  n185 = Or(x=w90, y=w89) -> (x .or. y?=→"L9" →"W8":bool)
  n186 = shared-variable "MGCC\\MGCC_FntStaMach_Functions.lvlib\\b_MGCC_FntStaMach_state_estimation_enable"() -> (→"State Estimation":bool)  [unwired: 1 in, 1 out]
  n187 = Greater?(x=w87, y=0.5) -> (0:w84:bool)
  n188 = Greater?(x=w88, y=0.5) -> (0:w83:bool)
  n189 = Or(x=w84, y=w83) -> (x .or. y?=→"L10":bool)
  n190 = shared-variable "BESS LC\\DNP3_Master_Station_OpalRT.lvlib\\DNP3_Master_Data_Variables.lvlib\\MS_Analog_Status.lvlib\\BESS-STATUS"() -> (w70:dbl)  [unwired: 1 in, 1 out]
  n191 = shared-variable "PV LC\\DNP3_Master_Station_Template.lvlib\\DNP3_Master_Data_Variables.lvlib\\MS_Analog_Status.lvlib\\PV-STATUS"() -> (w71:dbl)  [unwired: 1 in, 1 out]
  n192 = shared-variable "MGCC\\MGCC_EnergyMgmt_dataIO.lvlib\\b_MGCC_EnergyMgmt_Enable"() -> (→"Energy Mgmt.":bool)  [unwired: 1 in, 1 out]
  n193 = shared-variable "BESS LC\\DNP3_Master_Station_OpalRT.lvlib\\DNP3_Master_Data_Variables.lvlib\\MS_Analog_Status.lvlib\\BESS-STATUS"() -> (w247:dbl)  [unwired: 1 in, 1 out]
  n194 = shared-variable "BESS LC\\DNP3_Master_Station_OpalRT.lvlib\\DNP3_Master_Data_Variables.lvlib\\MS_Analog_Status.lvlib\\BESS-MAG"() -> ()  [unwired: 1 in, 2 out]
  n195 = shared-variable "MGCC\\MGCC_Commun_mainlib.lvlib\\b_MGCC_Commun_enable"() -> (→"Communication":bool)  [unwired: 1 in, 1 out]
  n196 = shared-variable "BESS LC\\DNP3_Master_Station_OpalRT.lvlib\\DNP3_Master_Data_Variables.lvlib\\MS_Analog_Status.lvlib\\BESS-SOC"() -> (→"Battery SOC" →"SOC Tank":dbl)  [unwired: 1 in, 1 out]
  n197 = shared-variable "MGCC\\MGCC_LoadFcst_dataIO.lvlib\\b_MGCC_LoadFcst_Enable"() -> (→"Load Forecasting":bool)  [unwired: 1 in, 1 out]
  n198 = shared-variable "MGCC\\MGCC.lvlib\\b_MGCC_DataLog_enable"() -> (→"Data Logging":bool)  [unwired: 1 in, 1 out]
  n199 = shared-variable "MGCC\\MGCC_MdlMgmt.lvlib\\b_MGCC_MdlMgmt_done"() -> (→"Model Mgmt.":bool)  [unwired: 1 in, 1 out]
  n200 = shared-variable "MGCC\\MGCC_BlkStart_Input.lvlib\\b_MGCC_BlkStart_Enable"() -> (→"Black Start":bool)  [unwired: 1 in, 1 out]
  n201 = shared-variable "MGCC\\MGCC_PVFcst_dataIO.lvlib\\b_MGCC_PVFcst_Enable"() -> (→"PV Forecasting":bool)  [unwired: 1 in, 1 out]
  n202 = shared-variable "MGCC\\MGCC_PQBal_Input.lvlib\\b_MGCC_PQBal_enable"() -> (→"PQ Balance":bool)  [unwired: 1 in, 1 out]
  n203 = shared-variable "MGCC\\DNP3_Master_Station_OpalRT.lvlib\\DNP3_Master_Data_Variables.lvlib\\MS_Analog_Status.lvlib\\S1011-status"() -> (w77:dbl)  [unwired: 1 in, 1 out]
  n204 = shared-variable "MGCC\\DNP3_Master_Station_OpalRT.lvlib\\DNP3_Master_Data_Variables.lvlib\\MS_Analog_Status.lvlib\\S1114-status"() -> (w76:dbl)  [unwired: 1 in, 1 out]
  n205 = Greater?(x=w247, y=0.5) -> (0:→"BESS LC":bool)
  n206 = Greater?(x=w71, y=0.5) -> (0:w69:bool)
  n207 = Greater?(x=w70, y=0.5) -> (0:w68:bool)
  n208 = Or(x=w69, y=w68) -> (x .or. y?=→"W9":bool)
  n209 = Greater?(x=w77, y=0.5) -> (0:w79:bool)
  n210 = Greater?(x=w76, y=0.5) -> (0:w78:bool)
  n211 = Or(x=w79, y=w78) -> (x .or. y?=→"W12" →"L11":bool)
  "Communication" <- TRUE ("Communication")
  "Resynchronization" <- TRUE ("Resynchronization")
  "Active power control" <- TRUE ("Active power control")
  "Reactive power control" <- TRUE ("Reactive power control")
  "Data Acquisition" <- TRUE ("Data Acquisition")
  "Communication" <- TRUE ("Communication")
  "Resynchronization" <- TRUE ("Resynchronization")
  "Active power control" <- TRUE ("Active power control")
  "Reactive power control" <- TRUE ("Reactive power control")
  "Data Acquisition" <- TRUE ("Data Acquisition")
